vi "delay.vi"(2 "delay":i16=500, 3 "x(n)":fxp<+/-,24,4>) -> (1 "x(n-N)":fxp<+/-,24,4> format="%.22g")   [LabVIEW 2023]
uses:
  <vilib>/Utility/error.llb/Clear Errors.vi
  <vilib>/rvi/Emulation/niFpgaSctlEmulationGetInTimedLoop.vi
  <vilib>/rvi/Memory/Memory_Emulation/nirvimemoryEmulation.vi
  <vilib>/rvi/Memory/Memory_Emulation/nirvimemoryFastEmulation.vi
  <vilib>/rvi/DataTransferAndStorage/Container/Common/niFpgaContainerGetUniqueNameForEmu.vi
  <vilib>/rvi/Memory/Memory_Emulation/niFpgaMemoryEmulationCacheClearOnFirstRun.vi
  <vilib>/rvi/Memory/Memory_Emulation/nirvimemoryEmulationManagerCache_MakeExclusive.vi
  <vilib>/rvi/Memory/Memory_Emulation/niFpgaMemoryEmulationValidateCache.vi
  <vilib>/rvi/Memory/Memory_Emulation/nirvimemoryEmulationManagerCache_InsertValue.vi
  <vilib>/rvi/Memory/Memory_Emulation/nirvimemoryEmulationManagerCache_ReleaseExclusive.vi
  <vilib>/rvi/Memory/Memory_Emulation/nirvimemoryEmulationManagerCache_GetValue.vi
  <vilib>/rvi/Emulation/niFpgaEmulationIsFPGAContextNoSignature.vi
  <vilib>/rvi/Memory/Memory_Emulation/nirvimemoryEmulationManagerCache_SetValue.vi
  <vilib>/rvi/Emulation/niFpgaSctlEmulationResourceMgr.vi
  <vilib>/rvi/DataTransferAndStorage/Container/Common/niFpgaContainerSetEmuInfo.vi
  <vilib>/rvi/eio/common/nirviEmuReportErrorAndStop.vi
  <vilib>/rvi/DataTransferAndStorage/Container/XNode/niFpgaContainer.xnode
  <vilib>/rvi/LocalResourceManager/LocalResourceManager.xnode
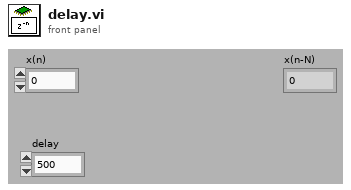
[diagram p1: front panel]
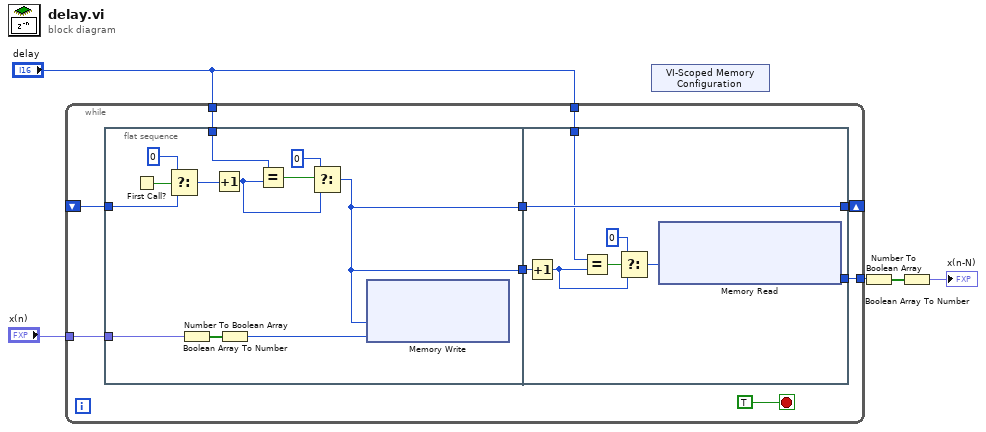
[diagram p0: block diagram]
diagram:
  n1 = while {
    tunnel: "x(n)" -> [w12]
    shift-right: [w11] -> _
    shift-left: _ -> [w9]
    tunnel: [w8] -> w2
    tunnel: "delay" -> [w7]
    tunnel: "delay" -> [w6]
    stop <- TRUE stop-if-true
    n2 = flat-sequence {
      tunnel: [w23] -> w14
      tunnel: w12 -> [w17]
      tunnel: [w23] -> w10
      tunnel: w9 -> [w21]
      tunnel: w7 -> [w18]
      tunnel: w14 -> [w30]
      tunnel: [w29] -> w11
      tunnel: w10 -> [w29]
      tunnel: [w28] -> w8
      tunnel: w6 -> [w27]
      frame #0 {
        n3 = First Call?() -> (First Call?: T/F=w22:bool)
        n4 = Select(t=i16 0, s=w22, f=w21) -> (s? t:f=w19:i16)
        n5 = Number To Boolean Array(number=w17) -> (Boolean array=w16:bool[])
        n6 = Increment(x=w19) -> (x+1=w24:i16)
        n7 = Boolean Array To Number(Boolean array=w16) -> (number=w15:i32)
        n8 = Equal?(x=w18, y=w24) -> (x = y?=w25:bool)
        n9 = Select(t=i16 0, s=w25, f=w24) -> (s? t:f=w23:i16)
        n10 = xnode ("Memory Write")("Address"=w23, "Data"=w15) -> ()  [unwired: 1 in, 1 out]
      }
      frame #1 {
        n11 = Increment(x=w30) -> (x+1=w33:i16)
        n12 = Equal?(x=w27, y=w33) -> (x = y?=w31:bool)
        n13 = Select(t=i16 0, s=w31, f=w33) -> (s? t:f=w34:i16)
        n14 = xnode ("Memory Read")("Address"=w34) -> ("Data"=w28:i32)  [unwired: 1 in, 1 out]
      }
    }
  }
  n15 = xnode "VI-Scoped Memory Configuration"() -> ()  [unwired: 1 out]
  n16 = Number To Boolean Array(number=w2) -> (Boolean array=w3:bool[])
  n17 = Boolean Array To Number(Boolean array=w3) -> (number=→"x(n-N)":fxp<+/-,24,4>)
